vi "User Plugin.vi"(5 "Initialize":bool, 8 "error in (no error)":errorcluster, 10 "ParamValues":sgl[](array[numeric]), 11 "DSI Reference":refnum<class "DCM-DSI-UserFuelTrimExample.lvclass">) -> (0 "error out":errorcluster, 3 "DSI Reference":refnum<class "DCM-DSI-UserFuelTrimExample.lvclass">, 4 "Results":T1[](array[typedef]), 6 "ParamNames":string[](array[string]))   [LabVIEW 2016, in "DCM-DSI-UserFuelTrimExample.lvclass"]
uses:
  DCM-DSI-UserFuelTrimExample.lvclass
  D:/PCG/Products/DCM/Software/DCM-DSI/Classes/DCM-DSI/DCM-DSI.lvclass
  Shared/Typedefs/UserParameter.ctl
  DCM-DSI/Read Channels.vi
  DCM-DSI/Read dt.vi
  Shared/DSI-Shared.lvlib
  DCM-DSI/DCM-DSI.lvclass
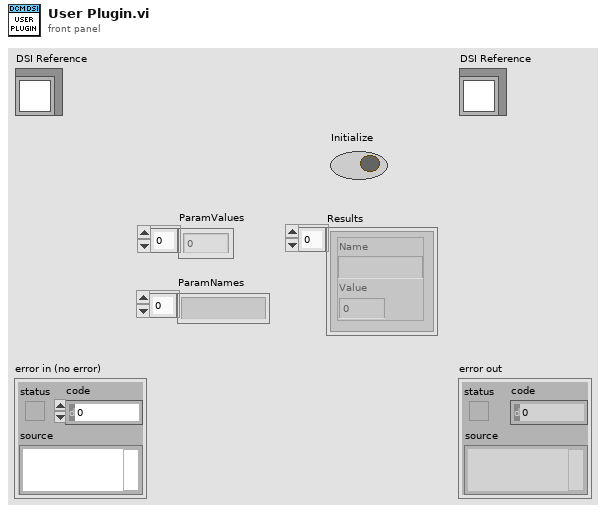
[diagram p1: front panel]
types:
  T1 = typedef "DSI-Shared.lvlib/UserParameter.ctl" = cluster{"Name":string, "Value":dbl}
  T2 = typedef "DSI-Shared.lvlib/Engine-Channel.ctl" = cluster{"Name":string, "Unit":string, "Value":sgl}
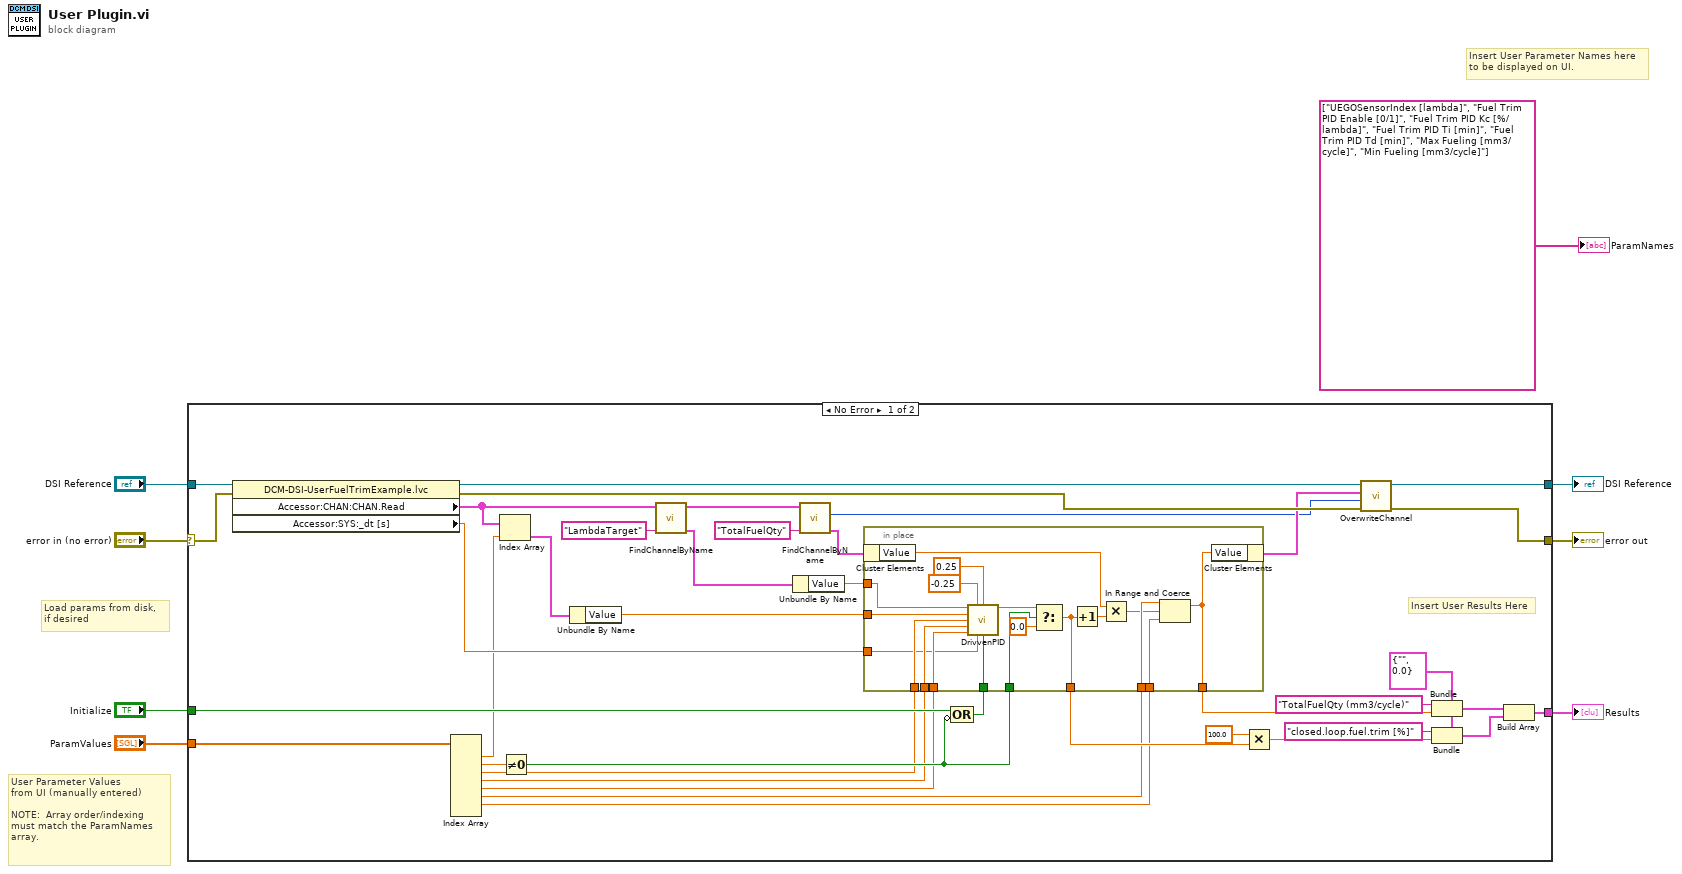
[diagram p0: block diagram]
diagram:
  # "Load params from disk,\nif desired"
  # "User Parameter Values\nfrom UI (manually entered)\n\nNOTE:  Array order/indexing\nmust match the ParamNames\narray."
  # "Insert User Parameter Names here\nto be displayed on UI."
  n1 = case shown="No Error" "error in (no error)" {
    selector: "error in (no error)" -> [w47 w68]
    tunnel: [w12 w68] -> w7
    tunnel: [w13 w67] -> w5
    tunnel: "DSI Reference" -> [w46 w67]
    tunnel: "Initialize" -> [w34 _]
    tunnel: "ParamValues" -> [w45 _]
    tunnel: [w44 _] -> w2
    frame No Error {
      w39 = T1 {"Name"="", "Value"=0.0} ("User Parameter")
      # "Insert User Results Here"
      n2 = property class="DCM-DSI-UserFuelTrimExample.lvc"(reference=w46, error in=w47) -> (reference out=w14:refnum<class "DCM-DSI-UserFuelTrimExample.lvclass">, error out=w11:errorcluster, "Accessor:CHAN:CHAN.Read"=w20:T2[], "Accessor:SYS:_dt [s]"=w25:sgl)
      n3 = Index Array(array=w45) -> (element #1=w15:sgl, element #2=w29:sgl, element #3=w28:sgl, element #4=w27:sgl, element #5=w26:sgl, element #6=w31:sgl, element #7=w30:sgl)  [unwired: 8 in, 1 out]
      n4 = Index Array(array=w20, index=w15) -> (element=w41:T2)
      n5 = Not Equal To 0?(x=w29) -> (x != 0?=w32:bool)
      n6 = Unbundle By Name(w41) -> ("Value"=w24:sgl)
      n7 = call "FindChannelByName.vi"("Name"="LambdaTarget", "CTRL.Channels in"=w20) -> ("Channel"=w18:T2, "CTRL.Channels out"=w19:T2[])  [unwired: 6 in, 2 out]
      n8 = Unbundle By Name(w18) -> ("Value"=w17:sgl)
      n9 = call "FindChannelByName.vi"("Name"="TotalFuelQty", "CTRL.Channels in"=w19) -> ("Channel"=w22:T2, "Index"=w9:i32)  [unwired: 6 in, 2 out]
      n10 = Compound Arithmetic op=OR(w34, invert w32) -> (w33:bool)
      n11 = in-place {
        in-place-border: [w66] -> w37
        in-place-border: w33 -> [w65]
        in-place-border: w32 -> [w64]
        in-place-border: w31 -> [w63]
        in-place-border: w30 -> [w62]
        in-place-border: [w48] -> w16
        in-place-border: w28 -> [w61]
        in-place-border: w27 -> [w60]
        in-place-border: w26 -> [w59]
        in-place-border: w25 -> [w58]
        in-place-border: w24 -> [w57]
        in-place-border: w17 -> [w49]
        n12 = in-place-cluster #1(w22) -> ("Value"=w50:sgl)
        n13 = call <vilib>:"DrivvenPID.vi"("Setpoint"=w49, "OutputLow"=sgl -0.25, "OutputHigh"=sgl 0.25, "ProcessVariable"=w57, "ProportionalGain (Kc)"=w61, "IntegralTime (Ti, min)"=w60, "DerivativeTime (Td, min)"=w59, "dt (s)"=w58, "Reinitialize? (F)"=w65) -> ("Output"=w55:sgl)  [unwired: 1 in, 5 out]
        n14 = Select(t=w55, s=w64, f=sgl 0.0) -> (s? t:f=w66:sgl)
        n15 = Increment(x=w66) -> (x+1=w51:sgl)
        n16 = Multiply(x=w50, y=w51) -> (x*y=w54:sgl)
        n17 = In Range and Coerce(upper limit=w63, x=w54, lower limit=w62) -> (coerced(x)=w48:sgl)  [unwired: 1 out]
        n18 = in-place-cluster #1("Value"=w48) -> (w10:T2)
      }
      n19 = Multiply(x=sgl 100.0, y=w37) -> (x*y=w35:sgl)
      n20 = call "OverwriteChannel.vi"("error in (no error)"=w11, "ChannelIndex"=w9, "Channel"=w10, "DCM-DSI-HW in"=w14) -> ("error out"=w12:errorcluster, "DCM-DSI-HW out"=w13:refnum<class "DCM-DSI-UserFuelTrimExample.lvclass">)  [unwired: 6 in]
      n21 = Bundle(cluster=w39, "Name"="TotalFuelQty (mm3/cycle)", "Value"=w16) -> (w42:T1)
      n22 = Bundle(cluster=w39, "Name"="closed.loop.fuel.trim [%]", "Value"=w35) -> (w38:T1)
      n23 = Build Array(w42, w38) -> (w44:T1[])
    }
    frame Error {
    }
  }
  "error out" <- w7
  "DSI Reference" <- w5
  "Results" <- w2
  "ParamNames" <- string[] ["UEGOSensorIndex [lambda]", "Fuel Trim PID Enable [0/1]", "Fuel Trim PID Kc [%/lambda]", "Fuel Trim PID Ti [min]", "Fuel Trim PID Td [min]", "Max Fueling [mm3/cycle]", "Min Fueling [mm3/cycle]"] ("ParamNames")
